vi "Call function.vi"(5 "log file path":string, 6 "cluster of jsons":T1, 7 "night dir":string, 8 "error in (no error)":errorcluster, 9 "Array":u16[][](array[numeric]), 10 "file name":string, 11 "Python Toolkit in":refnum<class "Python Toolkit.lvclass">) -> (0 "error out":errorcluster, 3 "Python Toolkit out":refnum<class "Python Toolkit.lvclass">)   [LabVIEW 2018, in "Python Toolkit.lvclass"]
doc: "Call a python function"
uses:
  Python Toolkit.lvclass
  Python Toolkit.lvclass/Python Toolkit.ctl
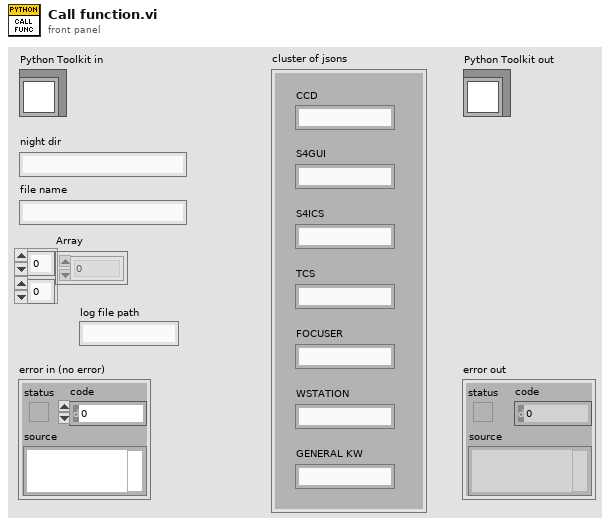
[diagram p1: front panel]
types:
  T1 = cluster{"CCD":string, "S4GUI":string, "S4ICS":string, "TCS":string, "FOCUSER":string, "WSTATION":string, "GENERAL KW":string}
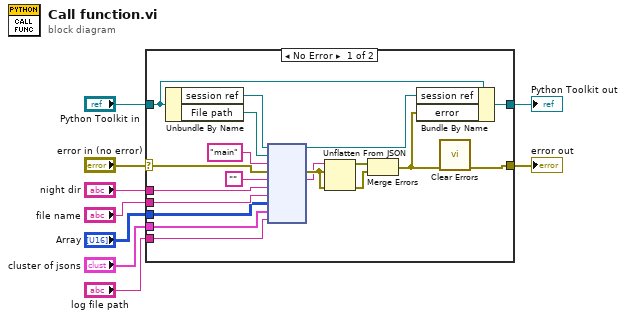
[diagram p0: block diagram]
diagram:
  n1 = case shown="No Error" "error in (no error)" {
    selector: "error in (no error)" -> [w28 w30]
    tunnel: [w10 w30] -> w8
    tunnel: [w26 w29] -> w6
    tunnel: "Python Toolkit in" -> [w27 w29]
    tunnel: "night dir" -> [w21 _]
    tunnel: "file name" -> [w20 _]
    tunnel: "Array" -> [w19 _]
    tunnel: "cluster of jsons" -> [w18 _]
    tunnel: "log file path" -> [w17 _]
    frame No Error {
      n2 = Unbundle By Name(w27) -> ("session ref"=w24:refnum<k35>, "File path"=w23:path)
      n3 = node(w24, w23, "main" ("function name"), w28, "", w21, w20, w19, w18, w17) -> (w25:refnum<k35>, w14:errorcluster, w13:string)  [unwired: 5 in, 2 out]
      n4 = Unflatten From JSON(JSON string=w13, type and defaults=w14, error in (no error)=w14) -> (value=w15:errorcluster, error out=w16:errorcluster)  [unwired: 4 in]
      n5 = Merge Errors(w15, w16) -> (w11:errorcluster)
      n6 = Bundle By Name(cluster=w27, "session ref"=w25, "error"=w11) -> (w26:refnum<class "Python Toolkit.lvclass">)
      n7 = call <vilib>:"Clear Errors.vi"("error in (no error)"=w11) -> ("error out"=w10:errorcluster)  [unwired: 5 in, 1 out]
    }
    frame Error {
    }
  }
  "error out" <- w8
  "Python Toolkit out" <- w6
